vi "AdvancedDemo.vi"() -> ()   [LabVIEW 2011]
uses:
  debug/TestDll.dll
  C:/Users/Behavior Room/Desktop/Kinect Mouse/DepthSense/FunctionPointerProxy/FunctionPointerProxy/obj/Release/FunctionPointerProxy.dll
  FunctionPointerProxy/obj/Release/FunctionPointerProxy.dll
panel:
  out "error out":errorcluster
  # "//Copyright (c) 2006 Bruno van Dooren\n//Permission is hereby granted, free of charge, to any person obtaining a copy\n//of this software and associated documentation files (the \"Software\"), to deal\n//in the Software without restriction, including without limitation the rights\n//to use, copy, modify, merge, publish, distribute, sublicense, and/or sell\n//copies of the Software, and to permit persons to whom the Software is\n//furnished to do so, subject to the following conditions:\n//The above copyright notice and this permission notice shall be included in all\n//copies or substantial portions of the Software.\n//THE SOFTWARE IS PROVIDED \"AS IS\", WITHOUT WARRANTY OF ANY KIND, EXPRESS OR\n//IMPLIED, INCLUDING BUT NOT LIMITED TO THE WARRANTIES OF MERCHANTABILITY,\n//FITNESS FOR A PARTICULAR PURPOSE AND NONINFRINGEMENT. IN NO EVENT SHALL THE\n//AUTHORS OR COPYRIGHT HOLDERS BE LIABLE FOR ANY CLAIM, DAMAGES OR OTHER\n//LIABILITY, WHETHER IN AN ACTION OF CONTRACT, TORT OR OTHERWISE, ARISING FROM,\n//OUT OF OR IN CONNECTION WITH THE SOFTWARE OR THE USE OR OTHER DEALINGS IN THE\n//SOFTWARE."
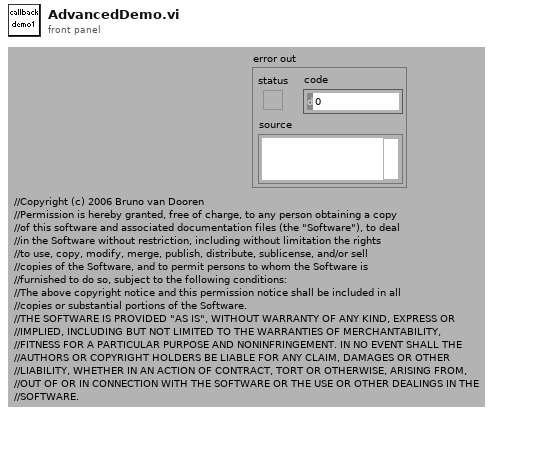
[diagram p1: front panel]
types:
  T1 = typedef "t_CallbackReferences.ctl" = cluster{"LV event callback ":refnum<k27>, "Proxy instance":refnum<k24>, "(*f)(...)":i32}
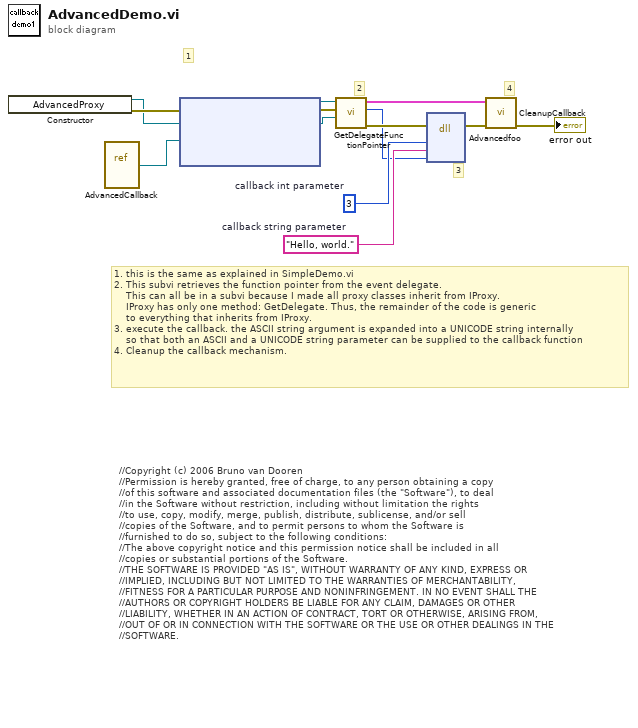
[diagram p0: block diagram]
diagram:
  w11 = "Hello, world."  # callback string parameter
  w12 = 3  # callback int parameter
  # "//Copyright (c) 2006 Bruno van Dooren\n//Permission is hereby granted, free of charge, to any person obtaining a copy\n//of this software and associated documentation files (the \"Software\"), to deal\n//in the Software without restriction, including without limitation the rights\n//to use, copy, modify, merge, publish, distribute, sublicense, and/or sell\n//copies of the Software, and to permit persons to whom the Software is\n//furnished to do so, subject to the following conditions:\n//The above copyright notice and this permission notice shall be included in all\n//copies or substantial portions of the Software.\n//THE SOFTWARE IS PROVIDED \"AS IS\", WITHOUT WARRANTY OF ANY KIND, EXPRESS OR\n//IMPLIED, INCLUDING BUT NOT LIMITED TO THE WARRANTIES OF MERCHANTABILITY,\n//FITNESS FOR A PARTICULAR PURPOSE AND NONINFRINGEMENT. IN NO EVENT SHALL THE\n//AUTHORS OR COPYRIGHT HOLDERS BE LIABLE FOR ANY CLAIM, DAMAGES OR OTHER\n//LIABILITY, WHETHER IN AN ACTION OF CONTRACT, TORT OR OTHERWISE, ARISING FROM,\n//OUT OF OR IN CONNECTION WITH THE SOFTWARE OR THE USE OR OTHER DEALINGS IN THE\n//SOFTWARE."
  # "1. this is the same as explained in SimpleDemo.vi\n2. This subvi retrieves the function pointer from the event delegate.\n    This can all be in a subvi because I made all proxy classes inherit from IProxy.\n    IProxy has only one method: GetDelegate. Thus, the remainder of the code is generic\n    to everything that inherits from IProxy.\n3. execute the callback. the ASCII string argument is expanded into a UNICODE string internally\n    so that both an ASCII and a UNICODE string parameter can be supplied to the callback function\n4. Cleanup the callback mechanism."
  # "3"
  # "4"
  # "2"
  # "1"
  n1 = constructor class="AdvancedProxy"() -> (reference out=w1:refnum<k24>, error out=w6:errorcluster)  [unwired: 3 in, 1 out]
  n2 = vi-ref "AdvancedCallback.vi"() -> ("vi reference"=w10:refnum<vi>)
  n3 = node(w6, w1, w10) -> (w9:refnum<k27>, w2:errorcluster)  [unwired: 2 in]
  n4 = call "GetDelegateFunctionPointer.vi"("target class"=w1, "error in (no error)"=w2, "event callback refnum"=w9) -> ("error out"=w8:errorcluster, "(*f)(...)"=w7:i32, "References"=w5:T1)  [unwired: 6 in]
  n5 = dll-call lib="D:/BlogFiles/LabVIEW/Callback_Interop/FunctionPointerProxy/debug/TestDll.dll" fn="Advancedfoo"(error in=w8, "i"=w12, "aString"=w11, "fPtr"=w7) -> (error out=w4:errorcluster)  [unwired: 6 in, 1 out]
  n6 = call "CleanupCallback.vi"("error in (no error)"=w4, "References"=w5) -> ("error out"=→"error out":errorcluster)  [unwired: 9 in]
